vi "Compute SEPL Wrapper.vi"(8 "error in (no error)":errorcluster, 11 "VI in":refnum<vi>) -> (0 "error out":errorcluster, 2 "Notebook String":string, 3 "Plot Name":string)   [LabVIEW 2019]
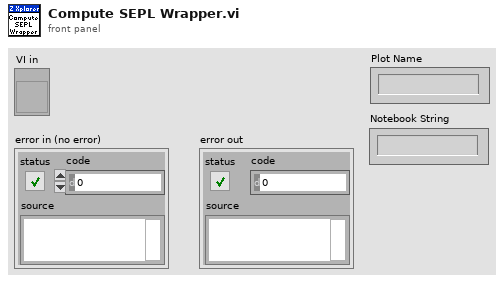
[diagram p1: front panel]
types:
  T1 = typedef "SEPL Parameters.ctl" = cluster{"Display Parameters":T2, "Phasor Parameters":T4, "Decay & IRF Parameters":T7, "Gate Parameters":T9, "Detector Parameters":T12}
  T2 = typedef "Phasor Explorer Display Parameters.ctl" = cluster{"# Points":i32, "Ramp Type":enum16{"Linear", "Logarithmic"}, "Type of Series":T3, "Min tau":dbl[unit], "Max tau":dbl[unit], "Include 0":bool, "Include Infinity":bool}
  T3 = typedef "Type of Series.ctl" = enum16{"1-Exp Decays", "Linear Combination of 1-Exp"}
  T4 = typedef "Phasor Explorer Phasor Parameters.ctl" = cluster{"Harmonic Frequency":dbl[unit], "Use f* = 1/D Frequency":bool, "Calibrated Phasor":bool, "Calibration Lifetime":dbl[unit], "Phasor Calculation":T5, "SEPL Type":T6, "# Gates":dbl, "Square Gate Width":dbl[unit], "Show Ticks":bool}
  T5 = typedef "Phasor Calculation Type.ctl" = enum16{"Direct Sum", "Analytical Formula"}
  T6 = typedef "SEPL Type.ctl" = enum16{"UC", "L_N", "L_N[W]", "L_X"}
  T7 = typedef "Phasor Explorer Decay Parameters.ctl" = cluster{"Lifetime":dbl[unit], "IRF Offset":dbl[unit], "IRF Period":dbl[unit], "Normalized Decays":bool, "IRF Model":T8, "IRF Parameter 1":dbl[unit]}
  T8 = typedef "IRF Model.ctl" = enum16{"Dirac", "Exponential"}
  T9 = typedef "Phasor Explorer Gate Parameters.ctl" = cluster{"First Gate Start":dbl[unit], "Use Gate Center":bool, "Gate Width":dbl[unit], "Gate Step":dbl[unit], "# Gates":dbl, "Gate Type":T10, "Edge Width":dbl[unit], "Top Slope":dbl[unit], "Reversed Sawtooth?":bool, "Analytical Computation":bool, "Integration":enum32{"Item 0", "Item 1"}, "Tolerance":dbl, "# Steps":dbl, "Type of User-defined Function":T11, "Use Gate Step":bool}
  T10 = typedef "Gate Type.ctl" = enum16{"Square", "Finite Edge Square", "Finite Edge, Tilted Top Square", "Triangle", "Sawtooth", "User-defined"}
  T11 = typedef "Type of User-defined Function.ctl" = enum16{"Gate", "IRF"}
  T12 = typedef "Phasor Explorer Detector Parameters.ctl" = cluster{"Frames/Image":i32, "Gates/Frame":i32, "Bits/Frame":i32, "Multiplicity":i32, "Incident Signal":dbl, "Poisson Signal":bool}
  T13 = typedef "Phasor Explorer Phasor Plot Info.ctl" = cluster{"Lifetime/Fraction Array":dbl[], "Phasor Explorer Parameters":T1, "Phase Lifetimes":dbl[], "Modulus Lifetimes":dbl[]}
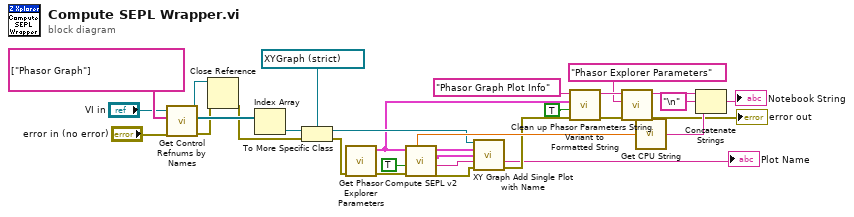
[diagram p0: block diagram]
diagram:
  n1 = call "Get Control Refnums by Names.vi"("error in"="error in (no error)", "Control Labels"=string[] ["Phasor Graph"], "VI  Ref"="VI in") -> ("error out"=w16:errorcluster, "Ctl Refnums"=w27:refnum<vi>[], "VI  Ref (out)"=w28:refnum<vi>)  [unwired: 5 in, 1 out]
  n2 = Close Reference(reference=w28, error in (no error)=w16) -> (error out=w15:errorcluster)
  n3 = Index Array(array=w27) -> (element=w25:refnum<vi>)  [unwired: 1 in]
  n4 = To More Specific Class(target class=refnum<vi> refnum ("Phasor Graph Refnum"), reference=w25, error in=w15) -> (specific class reference=w8:refnum<vi>, error out=w24:errorcluster)
  n5 = call "Get Phasor Explorer Parameters.vi"("Error In"=w24) -> ("Error Out"=w23:errorcluster, "Phasor Explorer Parameters"=w2:T1)  [unwired: 7 in, 2 out]
  n6 = call "Compute SEPL v2.vi"("Error In"=w23, "Compute Lifetime/Fraction Array"=TRUE, "Phasor Parameters"=w2) -> ("Error Out"=w10:errorcluster, "Plot Name"=w7:string, "Plot Metadata"=w4:T13, "Single Exponential Phasor Plot"=w6:cluster{"Array":dbl[], "Array":dbl[]}, "CPU (s)"=w14:dbl)  [unwired: 2 in, 2 out]
  n7 = call "XY Graph Add Single Plot with Name.vi"("XYGraph Ref in"=w8, "Plot"=w6, "Plot Metadata"=w4, "Plot Name (\"Plot\")"=w7, "error in (no error)"=w10) -> ("Plot Name"=→"Plot Name":string, "error out"=w9:errorcluster)  [unwired: 7 in, 2 out]
  n8 = call "Variant to Formatted String.vi"("Error In"=w9, "Hide Long Cluster Names (T)"=TRUE ("Hide Long Names (Cluster)"), "Variant"=w2, "Label"="Phasor Graph Plot Info") -> ("Error Out"=w19:errorcluster, "String"=w20:string)  [unwired: 6 in]
  n9 = call "Clean up Phasor Parameters String.vi"("Error In"=w19, "Cluster Label"="Phasor Explorer Parameters" ("regular expression"), "String in"=w20) -> ("Error Out"=→"error out":errorcluster, "String out"=w17:string)  [unwired: 7 in]
  n10 = call "Get CPU String.vi"("CPU (s)"=w14) -> ("String"=w12:string)  [unwired: 8 in]
  n11 = Concatenate Strings(w17, "\n" ("string"), w12) -> (→"Notebook String":string)
